vi "Actual Value Page.vi"(8 "error in (no error)":errorcluster, 11 "Node Ptr":T1 format="%.0x") -> (0 "error out":errorcluster)   [LabVIEW 2023, in "NI 272x Resistive Simulation Custom Device Configuration.lvlib"]
uses:
  NI 272x Resistive Simulation Custom Device Configuration.lvlib
  <vilib>/NI VeriStand/Custom Device API/Custom Device Item Ref.ctl
  Globals/Names.vi
  <vilib>/NI VeriStand/Custom Device API/Get Item Property (I32).vi
  <vilib>/NI VeriStand/Custom Device API/Custom Device API.lvlib
  NI 272x Resistive Simulation Custom Device Shared.lvlib
panel:
  out "Channel":i32
  out "Units":string
  in  "Header":cluster{"Section Name":string}={"Section Name"="Actual Hardware Channel Value"}
  in  "Description":string
  in  "Name":string
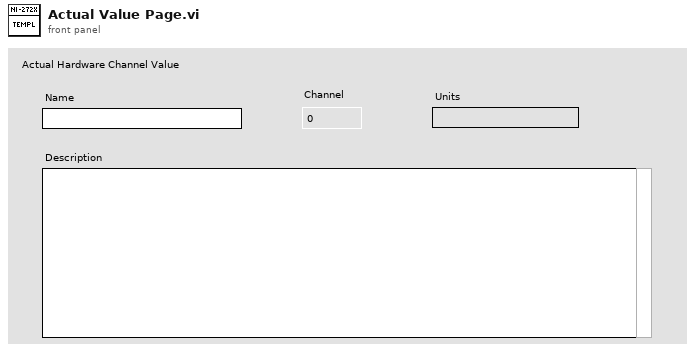
[diagram p1: front panel]
types:
  T1 = typedef "Custom Device API.lvlib/Custom Device Item Ref.ctl" = u64
  T2 = typedef "Custom Device API.lvlib/Custom Device Channel.ctl" = cluster{"Type":T3, "Units":string, "Default Value":dbl, "Faultable":bool, "Scalable":bool}
  T3 = typedef "Custom Device API.lvlib/Custom Device Channel Type.ctl" = enum16{"Input", "Output"}
  T4 = typedef "Custom Device API.lvlib/Custom Device Item Info.ctl" = cluster{"Name":string, "Is Channel":bool, "GUID":string, "Is Waveform":bool}
  T5 = typedef "Custom Device API.lvlib/Custom Device Commands.ctl" = enum16{"Default", "Item renamed", "Shutdown", "Dynamic button pressed"}
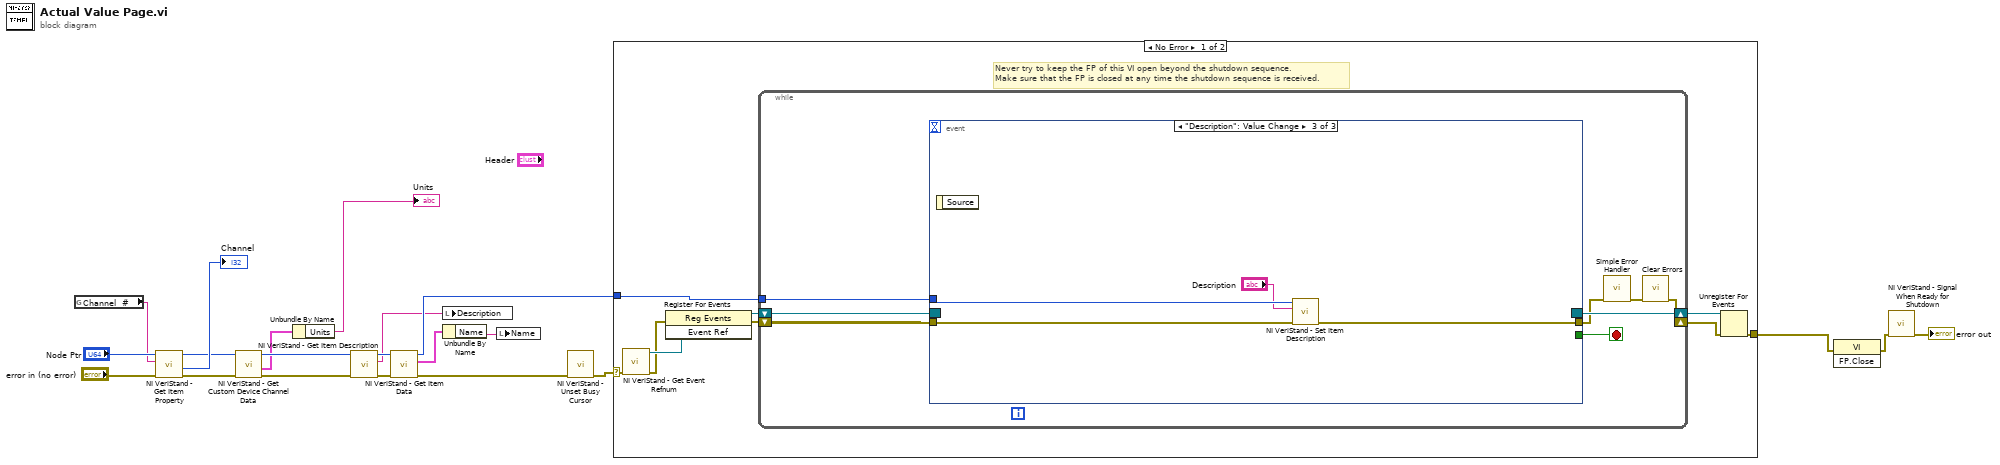
[diagram p0: block diagram]
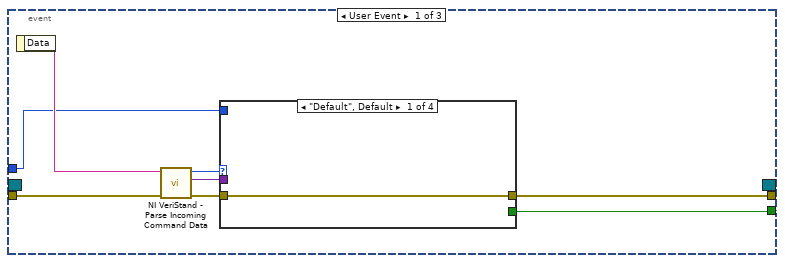
[diagram p2: hidden frame]
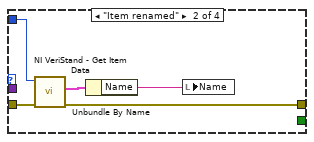
[diagram p3: hidden frame]
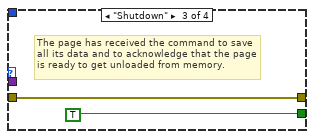
[diagram p4: hidden frame]
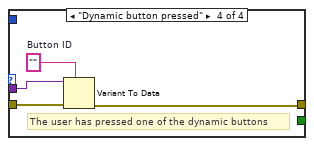
[diagram p5: hidden frame]
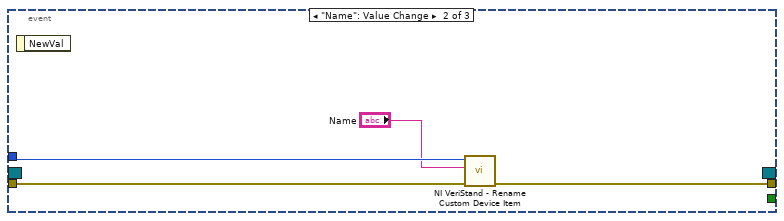
[diagram p6: hidden frame]
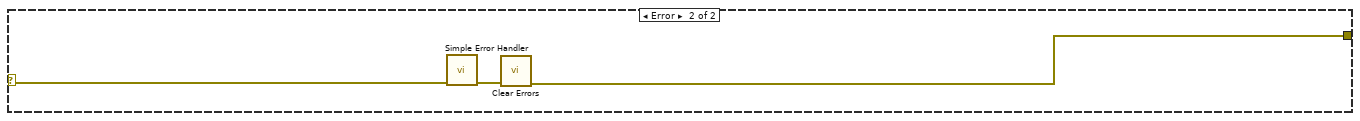
[diagram p7: hidden frame]
diagram:
  n1 = global read "Names.vi" "Channel  #"() -> (w7:string)
  n2 = call-poly <vilib>:"NI VeriStand - Get Item Property.vi"("error in (no error)"="error in (no error)", "Property Name"=w7, "Item Ref in"="Node Ptr") -> ("error out"=w9:errorcluster, "Value"=→"Channel":i32, "Item Ref out"=w4:T1)  [unwired: 5 in, 1 out]
  n3 = call <vilib>:"NI VeriStand - Get Custom Device Channel Data.vi"("error in (no error)"=w9, "Channel Ref in"=w4) -> ("error out"=w5:errorcluster, "Channel"=w2:T2, "Channel Ref out"=w3:T1)  [unwired: 4 in, 3 out]
  n4 = Unbundle By Name(w2) -> ("Units"=→"Units":string)
  n5 = call <vilib>:"NI VeriStand - Get Item Description.vi"("error in (no error)"=w5, "Item Ref in"=w3) -> ("error out"=w12:errorcluster, "Description"=w13:string, "Item Ref out"=w14:T1)  [unwired: 7 out]
  n6 = call <vilib>:"NI VeriStand - Get Item Data.vi"("error in (no error)"=w12, "Item Ref in"=w14) -> ("error out"=w15:errorcluster, "Item Info"=w11:T4, "Item Ref out"=w17:T1)  [unwired: 7 out]
  n7 = Unbundle By Name(w11) -> ("Name"=w10:string)
  n8 = local write "Description"(w13) -> ()
  n9 = local write "Name"(w10) -> ()
  n10 = call <vilib>:"NI VeriStand - Unset Busy Cursor.vi"("error in (no error)"=w15) -> ("error out"=w18:errorcluster)  [unwired: 10 out]
  n11 = case shown="No Error" w18 {
    selector: w18 -> [w23 w69]
    tunnel: [w28 w67] -> w21
    tunnel: w17 -> [w24 _]
    frame No Error {
      # "Never try to keep the FP of this VI open beyond the shutdown sequence.\nMake sure that the FP is closed at any time the shutdown sequence is received."
      n12 = call <vilib>:"NI VeriStand - Get Event Refnum.vi"("error in (no error)"=w23) -> ("error out"=w22:errorcluster, "Event Ref"=w27:refnum<user-event>)  [unwired: 9 out]
      n13 = register-events(error in=w22, w27) -> (reference out=w25:refnum<event-registration>, error out=w26:errorcluster)  [unwired: 1 in]
      n14 = while {
        tunnel: w24 -> [w34]
        shift-right: [w32] -> w29
        shift-left: w26 -> [w37]
        shift-right: [w38] -> w30
        shift-left: w25 -> [w36]
        stop <- w35 stop-if-true
        n15 = event shown="[2] \"Description\": Value Change" {
          selector: w36 -> [_ _ _]
          dyn-events: [_ _ _] -> w38
          timeout: _ -> [_ _ _]
          tunnel: w37 -> [w46 w62 w65]
          tunnel: [w42 _ _] -> w35
          tunnel: [w41 w59 w64] -> w31
          tunnel: w34 -> [w40 w61 w66]
          event User Event {
            n16 = event-data() -> ("Data"=w45:string)  [unwired: 1 out]
            n17 = call <vilib>:"NI VeriStand - Parse Incoming Command Data.vi"("error in (no error)"=w46, "Incoming data"=w45) -> ("error out"=w44:errorcluster, "Outgoing data"=w39:variant, "Action"=w43:T5)  [unwired: 7 out]
            n18 = case shown="\"Default\", Default" w43 {
              tunnel: w44 -> [w47 w52 w53 w58]
              tunnel: [_ _ TRUE _] -> w42
              tunnel: [w47 w49 w53 w55] -> w41
              tunnel: w40 -> [_ w51 _ _]
              tunnel: w39 -> [_ _ _ w57]
              frame "Default", Default {
              }
              frame "Item renamed" {
                n19 = call <vilib>:"NI VeriStand - Get Item Data.vi"("error in (no error)"=w52, "Item Ref in"=w51) -> ("error out"=w49:errorcluster, "Item Info"=w50:T4)  [unwired: 8 out]
                n20 = Unbundle By Name(w50) -> ("Name"=w48:string)
                n21 = local write "Name"(w48) -> ()
              }
              frame "Shutdown" {
                # "The page has received the command to save all its data and to acknowledge that the page is ready to get unloaded from memory."
              }
              frame "Dynamic button pressed" {
                w56 = ""  # Button ID
                # "The user has pressed one of the dynamic buttons"
                n22 = Variant To Data(error in=w58, type=w56, Variant=w57) -> (error out=w55:errorcluster)  [unwired: 1 out]
              }
            }
          }
          event "Name": Value Change {
            n23 = event-data() -> ()  [unwired: 2 out]
            n24 = call <vilib>:"NI VeriStand - Rename Custom Device Item.vi"("error in (no error)"=w62, "New Name"="Name", "Item Ref in"=w61) -> ("error out"=w59:errorcluster)  [unwired: 1 in, 7 out]
          }
          event "Description": Value Change {
            n25 = event-data() -> ()  [unwired: 2 out]
            n26 = call <vilib>:"NI VeriStand - Set Item Description.vi"("error in (no error)"=w65, "Description"="Description", "Item Ref in"=w66) -> ("error out"=w64:errorcluster)  [unwired: 8 out]
          }
        }
        n27 = call <vilib>:"Simple Error Handler.vi"("error in (no error)"=w31) -> ("error out"=w33:errorcluster)  [unwired: 1 in, 7 out]
        n28 = call <vilib>:"Clear Errors.vi"("error in (no error)"=w33) -> ("error out"=w32:errorcluster)  [unwired: 1 in, 5 out]
      }
      n29 = Unregister For Events(event registration refnum=w30, error in=w29) -> (error out=w28:errorcluster)
    }
    frame Error {
      n30 = call <vilib>:"Simple Error Handler.vi"("error in (no error)"=w69) -> ("error out"=w68:errorcluster)  [unwired: 1 in, 7 out]
      n31 = call <vilib>:"Clear Errors.vi"("error in (no error)"=w68) -> ("error out"=w67:errorcluster)  [unwired: 1 in, 5 out]
    }
  }
  n32 = invoke class="VI" method="FP.Close"(error in=w21) -> (error out=w20:errorcluster)  [unwired: 2 in, 2 out]
  n33 = call <vilib>:"NI VeriStand - Signal When Ready for Shutdown.vi"("error in (no error)"=w20) -> ("error out"=→"error out":errorcluster)  [unwired: 10 out]
